vi "Solve1.vi"(8 "Error In":errorcluster, 11 "object in":refnum<class "2021_17.lvclass">) -> (0 "Error Out":errorcluster, 2 "Result":u64, 3 "object out":refnum<class "2021_17.lvclass">)   [LabVIEW 2020, in "2021_17.lvclass"]
uses:
  2021_17.lvclass
  2021_17.lvclass/2021_17.ctl
panel:
  out "Array":i32[](array[numeric])
  out "X-Speeds":i32[](array[numeric])
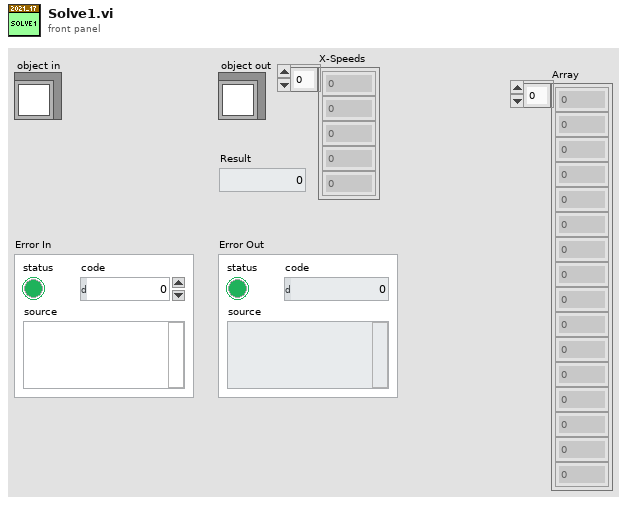
[diagram p1: front panel]
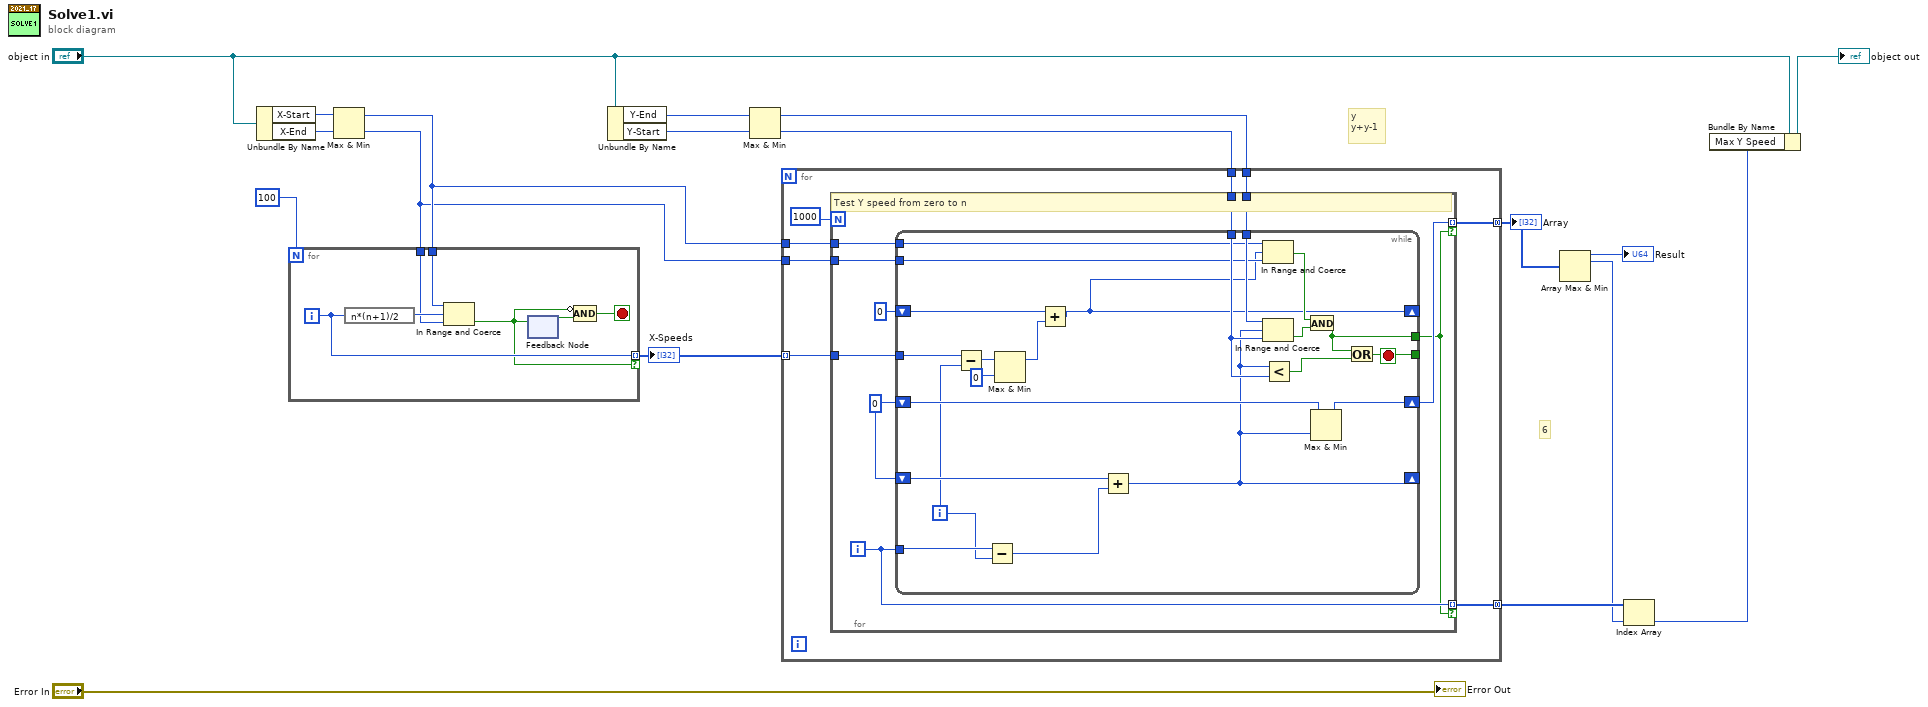
[diagram p0: block diagram]
diagram:
  # "6"
  # "y\ny+y-1"
  n1 = Unbundle By Name("object in") -> ("X-Start"=w14:i32, "X-End"=w13:i32)
  n2 = Max & Min(x=w14, y=w13) -> (max(x,y)=w8:i32, min(x,y)=w7:i32)
  n3 = for {
    N: 100 -> [_]
    tunnel: w7 -> [w24]
    tunnel: w8 -> [w23]
    tunnel: [w22] -> w16 mode=indexing if=w21
    i -> [w22]
    stop <- w19 stop-if-true
    n4 = expression code="n*(n+1)/2"(w22) -> (w25:i32)
    n5 = In Range and Coerce(upper limit=w23, x=w25, lower limit=w24) -> (In Range?=w21:bool)  [unwired: 1 out]
    n6 = feedback-in #1(w21) -> ()
    n7 = feedback #1() -> (w20:bool)  [unwired: 1 in]
    n8 = Compound Arithmetic op=AND(invert w21, w20) -> (w19:bool)
  }
  "X-Speeds" <- w16
  n9 = Unbundle By Name("object in") -> ("Y-End"=w12:i32, "Y-Start"=w11:i32)
  n10 = Max & Min(x=w12, y=w11) -> (max(x,y)=w10:i32, min(x,y)=w9:i32)
  n11 = for {
    tunnel: w16 -> [w29] mode=indexing
    tunnel: w10 -> [w32]
    tunnel: w9 -> [w31]
    tunnel: [w30] -> w6 mode=concatenating
    tunnel: w8 -> [w28]
    tunnel: w7 -> [w27]
    tunnel: [w26] -> w4 mode=concatenating
    n12 = for {
      N: 1000 -> [_]
      tunnel: w32 -> [w43]
      tunnel: w31 -> [w42]
      tunnel: [w37] -> w30 mode=indexing if=w34
      tunnel: w29 -> [w39]
      tunnel: w28 -> [w41]
      tunnel: w27 -> [w40]
      tunnel: [w35] -> w26 mode=indexing if=w34
      i -> [w35]
      w36 = 0
      # "Test Y speed from zero to n"
      n13 = while {
        tunnel: w43 -> [w65]
        tunnel: w42 -> [w64]
        tunnel: [w62] -> _
        tunnel: [w57] -> w34
        tunnel: w41 -> [w61]
        tunnel: w40 -> [w60]
        tunnel: w39 -> [w53]
        shift-right: [w54] -> _
        shift-left: 0 -> [w55]
        shift-right: [w48] -> w37
        shift-left: w36 -> [w49]
        shift-right: [w44] -> _
        shift-left: w36 -> [w56]
        tunnel: w35 -> [w47]
        i -> [w46]
        stop <- w62 stop-if-true
        n14 = Subtract(x=w53, y=w46) -> (x-y=w52:i32)
        n15 = Subtract(x=w47, y=w46) -> (x-y=w45:i32)
        n16 = Max & Min(x=w52, y=0) -> (max(x,y)=w51:i32)  [unwired: 1 out]
        n17 = Add(x=w55, y=w51) -> (x+y=w54:i32)
        n18 = Add(x=w56, y=w45) -> (x+y=w44:i32)
        n19 = In Range and Coerce(upper limit=w61, x=w54, lower limit=w60) -> (In Range?=w58:bool)  [unwired: 1 out]
        n20 = In Range and Coerce(upper limit=w65, x=w44, lower limit=w64) -> (In Range?=w59:bool)  [unwired: 1 out]
        n21 = Less?(x=w44, y=w64) -> (x < y?=w63:bool)
        n22 = And(x=w58, y=w59) -> (x .and. y?=w57:bool)
        n23 = Max & Min(x=w49, y=w44) -> (max(x,y)=w48:i32)  [unwired: 1 out]
        n24 = Or(x=w57, y=w63) -> (x .or. y?=w62:bool)
      }
    }
  }
  "Array" <- w6
  n25 = Array Max & Min(array=w6) -> (max value=→"Result":i32, max index (indices)=w3:i32)  [unwired: 2 out]
  n26 = Index Array(array=w4, index=w3) -> (element=w1:i32)
  n27 = Bundle By Name(cluster="object in", "Max Y Speed"=w1) -> (→"object out":refnum<class "2021_17.lvclass">)
  "Error Out" <- "Error In"
